vi "Configure Channel (Pulse Scale).vi"(0 "VISA resource name":refnum<visa-resource-name>, 1 "Channel (0001)":string="0001", 2 "Enable Channel (True)":bool=TRUE, 3 "Range (0 : Level)":i32(ring) items=["Level", "Contact"], 4 "Chattering filter (On)":bool=TRUE, 5 "error in (no error)":errorcluster, 7 "Span":T1={"Lower Span (0)"=0, "Upper Span (200000)"=200000} {"Upper Span (200000)" min=0 max=200000 step=1; "Lower Span (0)" min=0 max=200000 step=1}, 9 "Scaling":T2={"Floating point position (2)"=2, "Lower Scaling (0)"=0.0, "Upper Scaling (100)"=100.0, "Unit Character (\"\")"=""} {"Upper Scaling (100)" format="%_6g"; "Lower Scaling (0)" format="%_6g"; "Floating point position (2)" min=0 max=5 step=1}) -> (14 "VISA resource name out":refnum<visa-resource-name>, 15 "Channel":string, 19 "error out":errorcluster)   [LabVIEW 2020, in "Yokogawa GX Series.lvlib"]
doc: "Sets the input range of Pulse input channels.\n\nCommand: SRangePulse"
uses:
  <instrlib>/Yokogawa GX Series/Yokogawa GX Series.lvlib
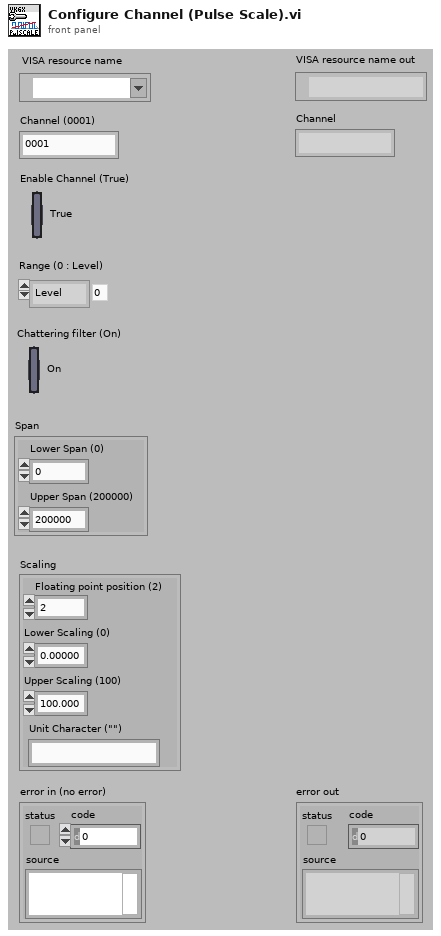
[diagram p1: front panel]
types:
  T1 = cluster{"Lower Span (0)":i32, "Upper Span (200000)":i32}
  T2 = cluster{"Floating point position (2)":i32, "Lower Scaling (0)":dbl, "Upper Scaling (100)":dbl, "Unit Character (\"\")":string}
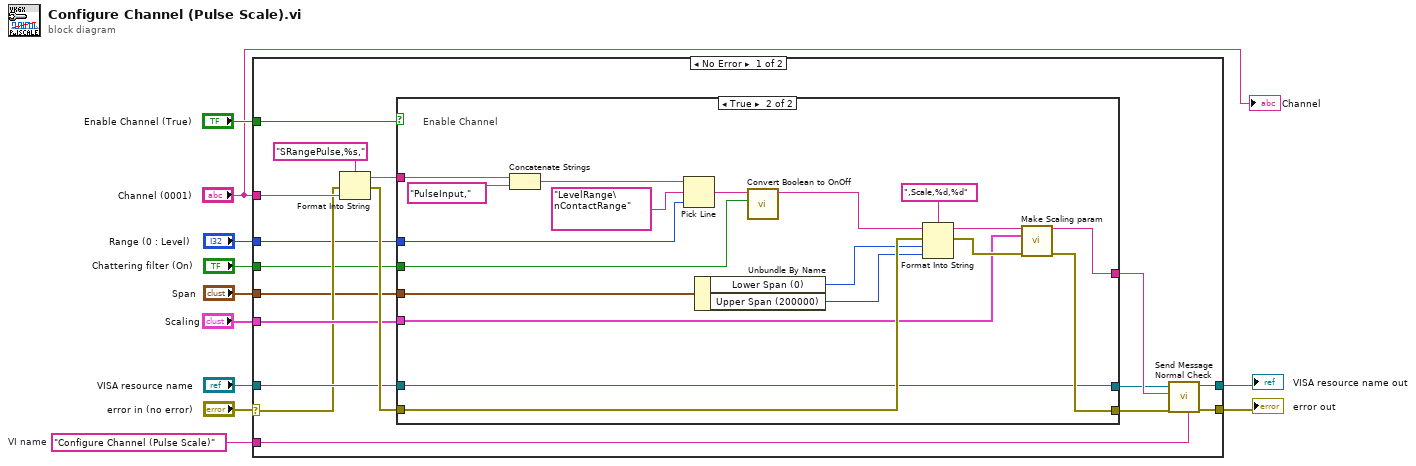
[diagram p0: block diagram]
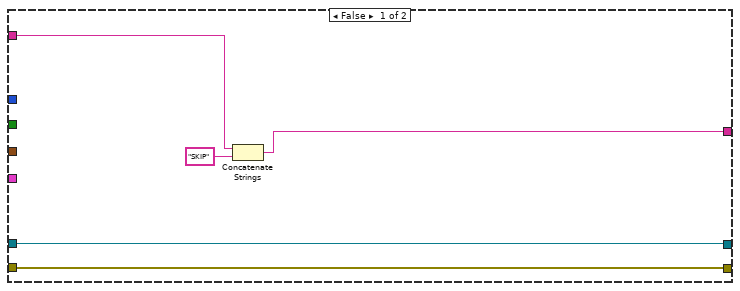
[diagram p2: hidden frame]
diagram:
  w10 = "Configure Channel (Pulse Scale)"  # VI name
  n1 = case shown="No Error" "error in (no error)" {
    selector: "error in (no error)" -> [w15 w53]
    tunnel: "Enable Channel (True)" -> [w25 _]
    tunnel: w10 -> [w22 _]
    tunnel: [w21 w54] -> w9
    tunnel: [w20 w53] -> w8
    tunnel: "VISA resource name" -> [w18 w54]
    tunnel: "Scaling" -> [w17 _]
    tunnel: "Channel (0001)" -> [w16 _]
    tunnel: "Span" -> [w14 _]
    tunnel: "Range (0 : Level)" -> [w13 _]
    tunnel: "Chattering filter (On)" -> [w12 _]
    frame No Error {
      n2 = Format Into String(format string="SRangePulse,%s,", error in=w15, w16) -> (resulting string=w26:string, error out=w27:errorcluster)  [unwired: 1 in]
      n3 = case shown="True" w25 {
        tunnel: w27 -> [w30 w51]
        tunnel: w26 -> [w31 w50]
        tunnel: [w30 w42] -> w24
        tunnel: [w32 w43] -> w23
        tunnel: [w29 w34] -> w19
        tunnel: w18 -> [w29 w34]
        tunnel: w17 -> [_ w44]
        tunnel: w14 -> [_ w41]
        tunnel: w13 -> [_ w38]
        tunnel: w12 -> [_ w36]
        frame False {
          n4 = Concatenate Strings(w31, "SKIP") -> (w32:string)
        }
        frame True {
          # "Enable Channel"
          n5 = Concatenate Strings(w50, "PulseInput,") -> (w40:string)
          n6 = Pick Line(string ("")=w40, multi-line string="LevelRange\nContactRange", line index=w38) -> (output string=w37:string)
          n7 = Unbundle By Name(w41) -> ("Lower Span (0)"=w48:i32, "Upper Span (200000)"=w47:i32)
          n8 = call <instrlib>:"Convert Boolean to OnOff.vi"("On/Off"=w36, "Initial String (\"\")"=w37) -> ("Resulting String"=w35:string)  [unwired: 9 in]
          n9 = Format Into String(format string=",Scale,%d,%d", initial string=w35, error in=w51, w48, w47) -> (resulting string=w46:string, error out=w45:errorcluster)
          n10 = call <instrlib>:"Make Scaling param.vi"("String (\"\")"=w46, "Scaling"=w44, "error in (no error)"=w45) -> ("String After"=w43:string, "error out"=w42:errorcluster)  [unwired: 11 in]
        }
      }
      n11 = call <instrlib>:"Send Message Normal Check.vi"("Source (\"\")"=w22, "error in (no error)"=w24, "Send Message (\"\")"=w23, "VISA resource name"=w19) -> ("error out"=w20:errorcluster, "VISA resource name out"=w21:refnum<visa-resource-name>)  [unwired: 2 in, 4 out]
    }
    frame Error {
    }
  }
  "error out" <- w8
  "VISA resource name out" <- w9
  "Channel" <- "Channel (0001)"
